vi "GetEvtReports.vi"(8 "error in (no error)":errorcluster, 11 "EventFromCSVPlugin in":refnum<class "EventFromCSVPlugin.lvclass">) -> (0 "error out":errorcluster, 3 "EventFromCSVPlugin out":refnum<class "EventFromCSVPlugin.lvclass">)   [LabVIEW 2014, in "EventPlugins.lvlib" / "EventFromCSVPlugin.lvclass"]
uses:
  EventFromCSVPlugin.lvclass
  Framework/Config_class/Config.lvclass/Config.ctl
  EventPluginBaseClass/TypeDefs/clEvtReportArray.ctl
  EventPluginBaseClass/TypeDefs/clEvtReport.ctl
  EventPluginBaseClass/EventPluginBaseClass.lvclass/EventPluginBaseClass.ctl
  EventPluginBaseClass/Accessors/Read BusNumber.vi
  Framework/Config_class/Accessors/Read PARTF Root Directory.vi
  EventPluginBaseClass/Accessors/Read EvtParams.vi
  <vilib>/Utility/error.llb/Error Cluster From Error Code.vi
  <vilib>/Utility/file.llb/Read From Spreadsheet File (DBL).vi
  <vilib>/ErrorRing/Error Ring.xnode
  EventPluginBaseClass/EventPluginBaseClass.lvclass
  Framework/Config_class/Config.lvclass
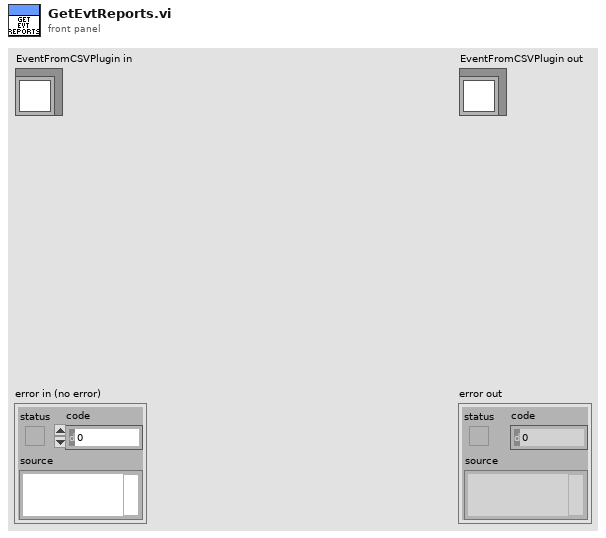
[diagram p1: front panel]
types:
  T1 = typedef "EventPlugins.lvlib/EventPluginBaseClass.lvclass/clEvtReportArray.ctl" = T2[]
  T2 = typedef "EventPlugins.lvlib/EventPluginBaseClass.lvclass/clEvtReport.ctl" = cluster{"Timestamp":dbl, "Synx":cdb[], "Freq":dbl, "ROCOF":dbl, "ID":i16}
  T3 = typedef "Framework.lvlib/Config.lvclass/RootDir.ctl" = cluster{"pathRootDir":path, "btnOutPath":bool, "OutDir":string, "btnOpenOutputDir":bool, "ScriptDir":string, "btnOpenScriptDir":bool, "TestDir":string, "btnOpenTestDir":bool}
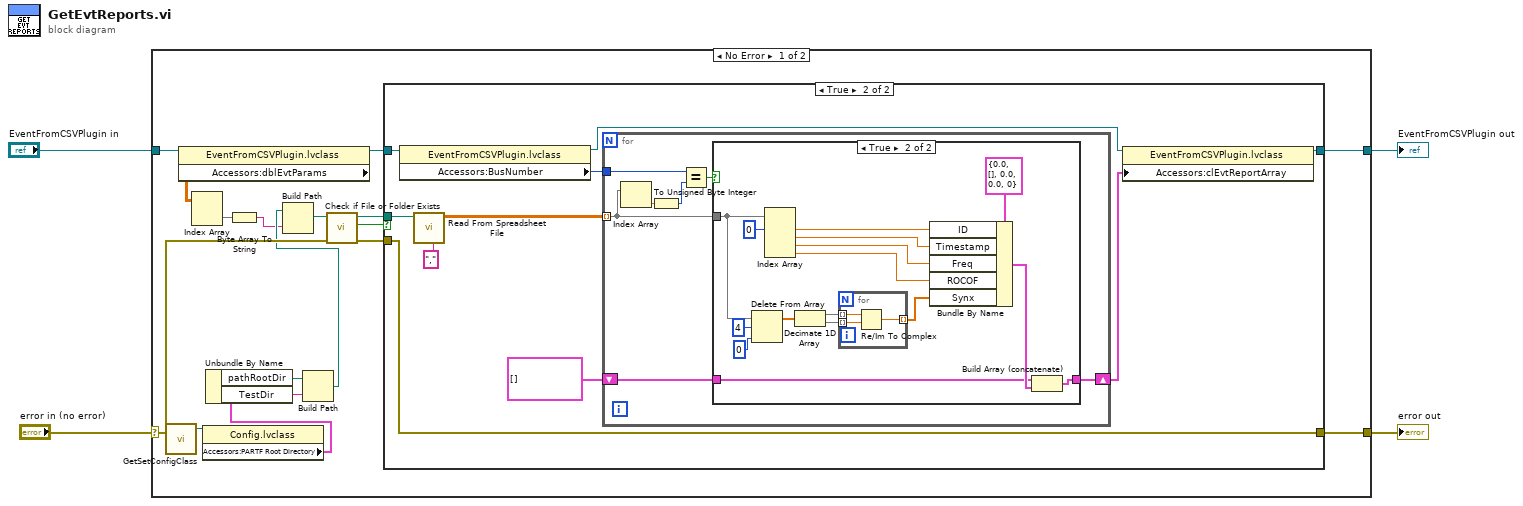
[diagram p0: block diagram]
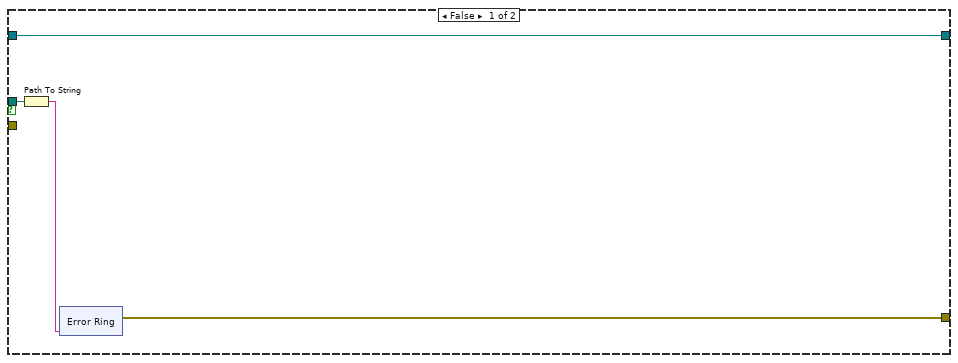
[diagram p2: hidden frame]
diagram:
  n1 = case shown="No Error" "error in (no error)" {
    selector: "error in (no error)" -> [w13 w71]
    tunnel: [w12 w71] -> w3
    tunnel: "EventFromCSVPlugin in" -> [w21 w70]
    tunnel: [w14 w70] -> w1
    frame No Error {
      n2 = call "GetSetConfigClass.vi"() -> ("Ref out"=w11:refnum<class "Config.lvclass">)  [unwired: 11 in]
      n3 = property class="EventFromCSVPlugin.lvclass"(reference=w21) -> (reference out=w15:refnum<class "EventFromCSVPlugin.lvclass">, "Accessors:dblEvtParams"=w20:dbl[][])  [unwired: 1 in, 1 out]
      n4 = Index Array(array=w20) -> (element=w19:dbl[])  [unwired: 2 in]
      n5 = property class="Config.lvclass"(reference=w11) -> ("Accessors:PARTF Root Directory"=w10:T3)  [unwired: 1 in, 2 out]
      n6 = Unbundle By Name(w10) -> ("pathRootDir"=w9:path, "TestDir"=w8:string)
      n7 = Byte Array To String(unsigned byte array=w19) -> (string=w5:string)
      n8 = Build Path(base path=w9, name or relative path=w8) -> (appended path=w6:path)
      n9 = Build Path(base path=w6, name or relative path=w5) -> (appended path=w7:path)
      n10 = call <vilib>:"Check if File or Folder Exists.vi"("error in (no error)"=w13, "path"=w7) -> ("error out"=w17:errorcluster, "file or folder exists?"=w18:bool, "dup path"=w16:path)  [unwired: 7 in]
      n11 = case shown="True" w18 {
        tunnel: w17 -> [_ w33]
        tunnel: w16 -> [w25 w42]
        tunnel: [w23 w33] -> w12
        tunnel: w15 -> [w22 w40]
        tunnel: [w22 w34] -> w14
        frame False {
          n12 = Path To String(path=w25) -> (string=w24:string)
          n13 = xnode "Error Ring"("parameter 0"=w24) -> ("error out"=w23:errorcluster)
        }
        frame True {
          n14 = property class="EventFromCSVPlugin.lvclass"(reference=w40) -> (reference out=w36:refnum<class "EventFromCSVPlugin.lvclass">, "Accessors:BusNumber"=w38:u8)  [unwired: 1 in, 1 out]
          n15 = call-poly <vilib>:"Read From Spreadsheet File.vi"("delimiter (\\t)"="," ("delimiter (\\t)"), "file path (dialog if empty)"=w42) -> ("all rows"=w39:dbl[][])  [unwired: 5 in, 4 out]
          n16 = for {
            tunnel: w39 -> [w46] mode=indexing
            tunnel: w38 -> [w45]
            shift-right: [w43] -> w35
            shift-left: T1 [] ("clEvtReportArray") -> [w44]
            n17 = Index Array(array=w46) -> (element=w49:dbl)  [unwired: 1 in]
            n18 = To Unsigned Byte Integer(number=w49) -> (unsigned 8bit integer=w48:u8)
            n19 = Equal?(x=w45, y=w48) -> (x = y?=w47:bool)
            n20 = case shown="True" w47 {
              tunnel: w46 -> [_ w64]
              tunnel: w44 -> [w50 w51]
              tunnel: [w50 w53] -> w43
              frame False {
              }
              frame True {
                n21 = Delete From Array(array=w64, length=4, index=0) -> (array with subset deleted=w61:dbl[])  [unwired: 1 out]
                n22 = Index Array(array=w64, index #1=0 ("index")) -> (element #1=w58:dbl, element #2=w57:dbl, element #3=w56:dbl, element #4=w55:dbl)  [unwired: 3 in]
                n23 = Decimate 1D Array(w61) -> (w60:dbl[], w59:dbl[])
                n24 = for {
                  tunnel: w60 -> [w69] mode=indexing
                  tunnel: w59 -> [w68] mode=indexing
                  tunnel: [w67] -> w54 mode=indexing
                  n25 = Re/Im To Complex(1:w68, 2:w69) -> (0:w67:cdb)
                }
                n26 = Bundle By Name(cluster=T2 {"Timestamp"=0.0, "Synx"=[], "Freq"=0.0, "ROCOF"=0.0, "ID"=0} ("clEvtReport"), "ID"=w58, "Timestamp"=w57, "Freq"=w56, "ROCOF"=w55, "Synx"=w54) -> (w52:T2)
                n27 = Build Array (concatenate)(w51, w52) -> (w53:T1)
              }
            }
          }
          n28 = property class="EventFromCSVPlugin.lvclass"(reference=w36, "Accessors:clEvtReportArray"=w35) -> (reference out=w34:refnum<class "EventFromCSVPlugin.lvclass">)  [unwired: 1 in, 1 out]
        }
      }
    }
    frame Error {
    }
  }
  "error out" <- w3
  "EventFromCSVPlugin out" <- w1
